vi "Verify Indents.vi"(10 "Tree Arr":T1(array[cluster]), 11 "Properties for Tree Out 2":T2(array[cluster])) -> (2 "First Fail Index":i32, 3 "Indents OK":bool)   [LabVIEW 2023]
doc: "Confirm that indents are legal (first is level 0, subsequent are equal to curremt, current+1, or less than current)\n\nTakes either of two types of input arrays."
panel:
  out "First Item 0?":bool
  out "Remaining items OK?":bool[](array[boolean])
  out "Indents":u16[](array[numeric])
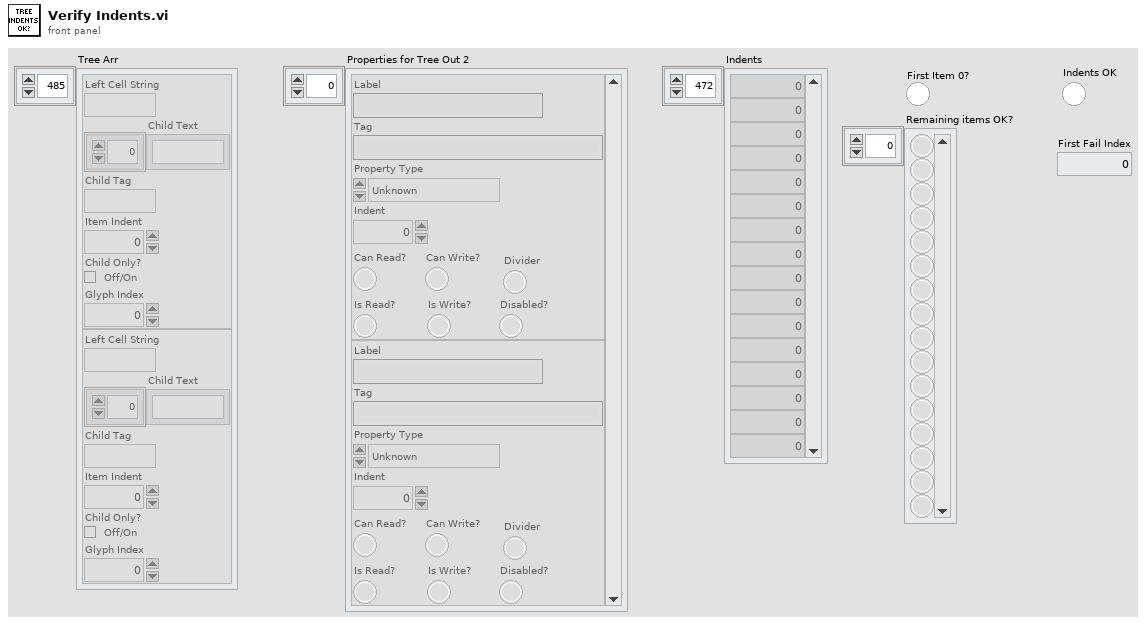
[diagram p1: front panel]
types:
  T1 = cluster{"Left Cell String":string, "Child Text":string[], "Child Tag":string, "Item Indent":i32, "Child Only?":bool, "Glyph Index":i32}[]
  T2 = cluster{"Label":string, "Tag":string, "Property Type":enum16{"Unknown", "Base", "Scripting", "Private", "Deprecated"}, "Indent":u16, "Can Read?":bool, "Can Write?":bool, "Is Read?":bool, "Is Write?":bool, "Disabled?":bool, "Divider":bool}[]
  T3 = cluster{"Left Cell String":string, "Child Text":string[], "Child Tag":string, "Item Indent":i32, "Child Only?":bool, "Glyph Index":i32}
  T4 = cluster{"Label":string, "Tag":string, "Property Type":enum16{"Unknown", "Base", "Scripting", "Private", "Deprecated"}, "Indent":u16, "Can Read?":bool, "Can Write?":bool, "Is Read?":bool, "Is Write?":bool, "Disabled?":bool, "Divider":bool}
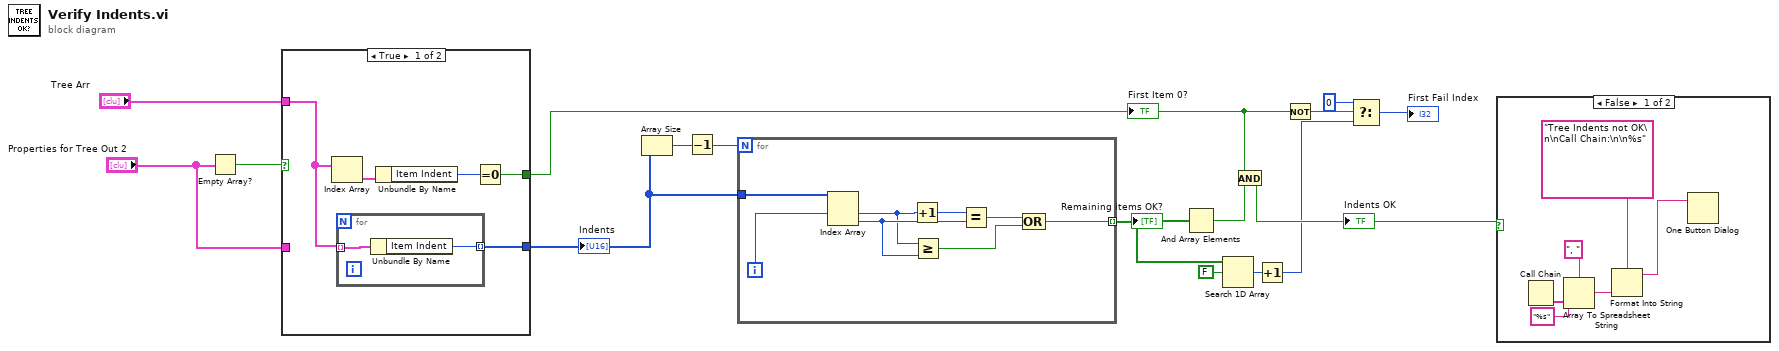
[diagram p0: block diagram]
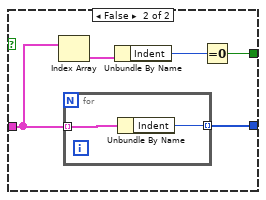
[diagram p2: hidden frame]
diagram:
  n1 = Empty Array?(array="Properties for Tree Out 2") -> (empty?=w9:bool)
  n2 = case shown="True" w9 {
    tunnel: [w19 w26] -> w14
    tunnel: [w18 w25] -> w6
    tunnel: "Properties for Tree Out 2" -> [_ w24]
    tunnel: "Tree Arr" -> [w17 _]
    frame True {
      n3 = Index Array(array=w17) -> (element=w20:T3)  [unwired: 1 in]
      n4 = for {
        tunnel: w17 -> [w23] mode=indexing
        tunnel: [w22] -> w19 mode=indexing
        n5 = Unbundle By Name(w23) -> ("Item Indent"=w22:i32)
      }
      n6 = Unbundle By Name(w20) -> ("Item Indent"=w21:i32)
      n7 = Equal To 0?(x=w21) -> (x = 0?=w18:bool)
    }
    frame False {
      n8 = Index Array(array=w24) -> (element=w27:T4)  [unwired: 1 in]
      n9 = for {
        tunnel: w24 -> [w30] mode=indexing
        tunnel: [w29] -> w26 mode=indexing
        n10 = Unbundle By Name(w30) -> ("Indent"=w29:u16)
      }
      n11 = Unbundle By Name(w27) -> ("Indent"=w28:u16)
      n12 = Equal To 0?(x=w28) -> (x = 0?=w25:bool)
    }
  }
  "Indents" <- w14
  "First Item 0?" <- w6
  n13 = Array Size(array=w14) -> (size(s)=w16:i32)
  n14 = Decrement(x=w16) -> (x-1=w15:i32)
  n15 = for {
    N: w15 -> [_]
    tunnel: w14 -> [w38]
    tunnel: [w33] -> w8 mode=indexing
    i -> [w37]
    n16 = Index Array(array=w38, index #1=w37) -> (element #1=w31:i32, element #2=w32:i32)  [unwired: 1 in]
    n17 = Increment(x=w31) -> (x+1=w36:i32)
    n18 = Greater Or Equal?(x=w31, y=w32) -> (x >= y?=w34:bool)
    n19 = Equal?(x=w36, y=w32) -> (x = y?=w35:bool)
    n20 = Compound Arithmetic op=OR(w35, w34) -> (w33:bool)
  }
  "Remaining items OK?" <- w8
  n21 = And Array Elements(Boolean array=w8) -> (logical AND=w13:bool)
  n22 = Search 1D Array(1D array=w8, element=FALSE) -> (index of element=w5:i32)  [unwired: 1 in]
  n23 = And(x=w6, y=w13) -> (x .and. y?=w12:bool)
  "Indents OK" <- w12
  n24 = Increment(x=w5) -> (x+1=w2:i32)
  n25 = Not(x=w6) -> (.not. x?=w1:bool)
  n26 = Select(t=0, s=w1, f=w2) -> (s? t:f=→"First Fail Index":i32)
  n27 = case shown="False" w12 {
    frame False {
      n28 = Call Chain() -> (call chain=w43:string[])
      n29 = Array To Spreadsheet String(delimiter (Tab)=", ", array=w43, 3:"%s" ("format string")) -> (spreadsheet string=w42:string)
      n30 = Format Into String(format string="Tree Indents not OK\n\nCall Chain:\n\n%s", w42) -> (resulting string=w39:string)  [unwired: 2 in, 1 out]
      n31 = One Button Dialog(message=w39) -> ()  [unwired: 1 in, 1 out]
    }
    frame True {
    }
  }
